vi "Main.vi"() -> ()   [LabVIEW 2018]
uses:
  States.ctl
panel:
  out "Minimalna waga pełnego akwarium":dbl format="%.2f"
  out "Współrzędne Y":dbl[](array[numeric]) format="%.2g"
  out "Współrzędne X":dbl[](array[numeric]) format="%.2g"
  out "Mocne punkty kompozycji":cluster{dbl[], dbl[]}(graph)
  out "Wykres pH wody w ciągu 23 dni":dbl[](graph)
  out "Waga pustego\n    akwarium":dbl format="%.2f"
  out "Rodzaje odczynów w\n       ciągu 23 dni":string[](array[string])
  out "Objętość brutto":dbl format="%.2g"
  out "Objętość netto":dbl format="%.2g"
  out "Wymagana ilość wody":dbl format="%.2g"
  out "pH wody w ciągu 23 dni":dbl[](array[numeric]) format="%.2f"
  in  "Wysokość":dbl=100.0 min=0.0
  in  "Długość":dbl=50.0 min=0.0
  in  "Szerokość":dbl=50.0 min=0.0
  in  "Grubość szyby":dbl=8.0 min=0.0
  in  "Zatrzymaj program":bool
  in  "Rysuj wykres mocnych punktów":bool
  in  "Policz wagę pustego\n        akwarium":bool
  in  "Rozpocznij symulację":bool
  # "Informacje zwrotne"
  # "Wprowadź dane \ndotyczące akwarium"
  # "l"
  # "cm"
  # "l"
  # "cm"
  # "l"
  # "cm"
  # "mm"
  # "kg"
  # "kg"
  # "Współrzędne punktów"
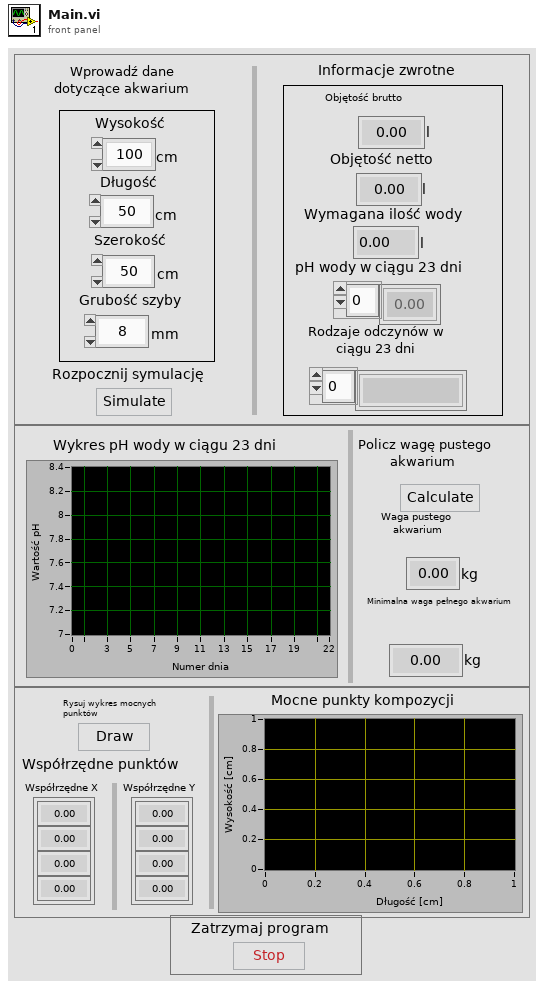
[diagram p1: front panel]
types:
  T1 = typedef "States.ctl" = enum16{"Init", "Idle", "Stop", "Simulate", "Calculate", "Draw"}
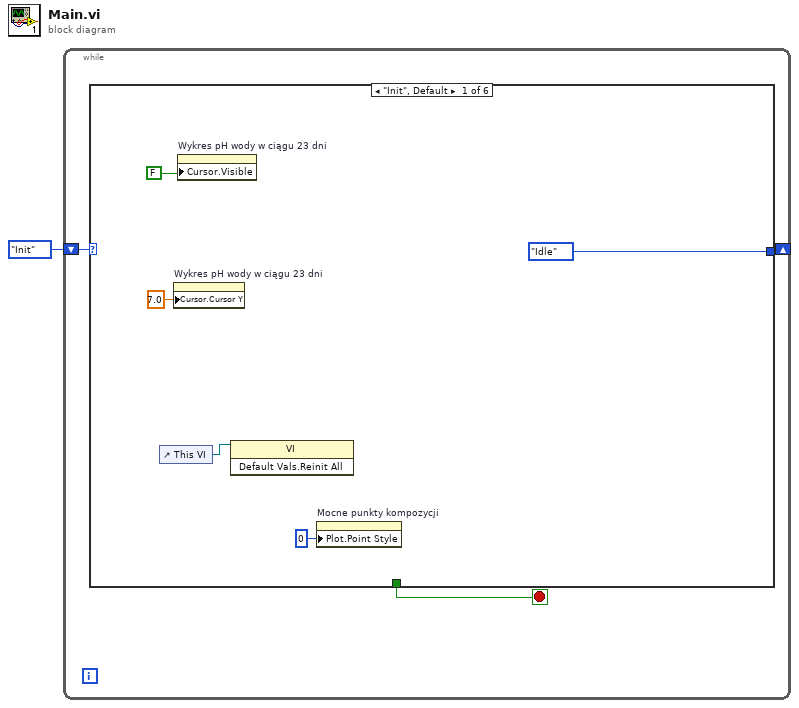
[diagram p0: block diagram]
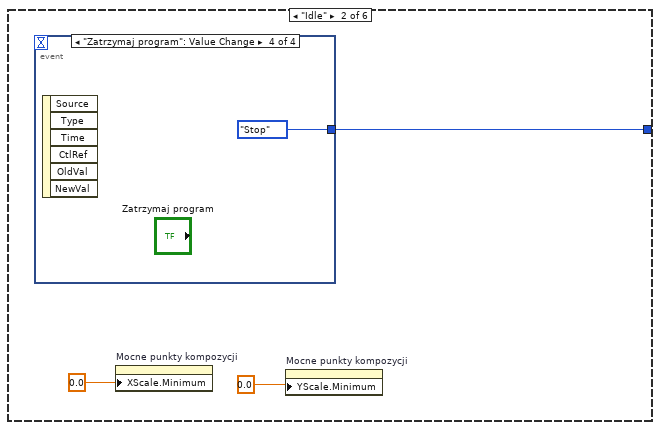
[diagram p2: hidden frame]
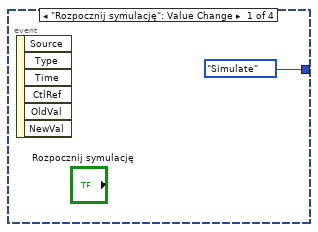
[diagram p3: hidden frame]
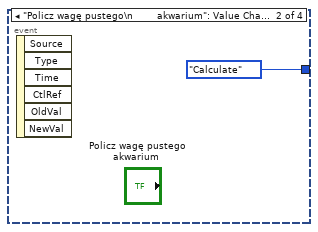
[diagram p4: hidden frame]
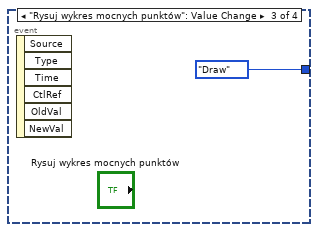
[diagram p5: hidden frame]
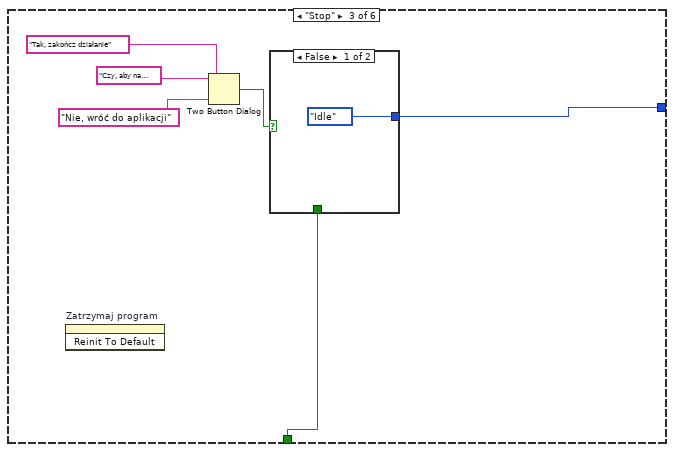
[diagram p6: hidden frame]
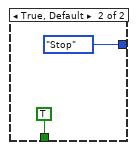
[diagram p7: hidden frame]
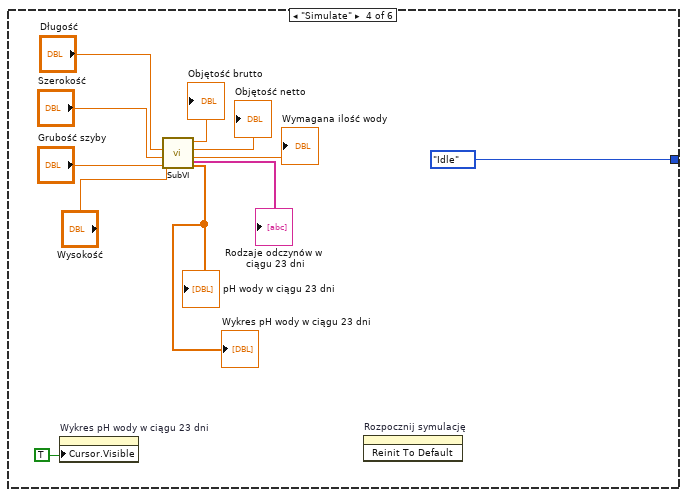
[diagram p8: hidden frame]
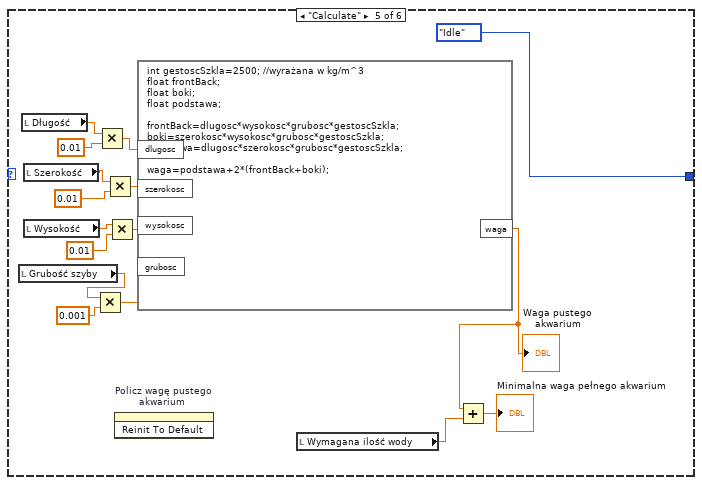
[diagram p9: hidden frame]
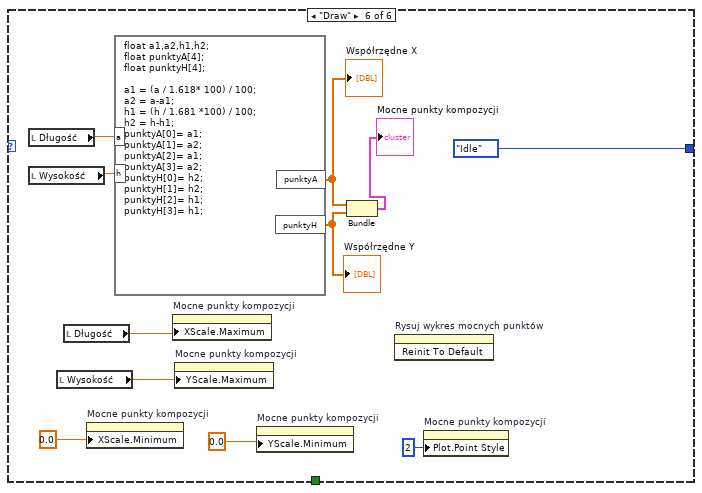
[diagram p10: hidden frame]
diagram:
  n1 = while {
    shift-right: [w2] -> _
    shift-left: States."Init" -> [w4]
    stop <- w3 stop-if-true
    n2 = case shown="\"Init\", Default" w4 {
      tunnel: [_ _ w18 _ _ _] -> w3
      tunnel: [States."Idle" w12 w17 States."Idle" States."Idle" States."Idle"] -> w2
      frame "Init", Default {
        n3 = control-ref of="This VI"() -> (w7:refnum<vi>)
        n4 = property on="Wykres pH wody w ciągu 23 dni" class="WFGraph (strict)"("Cursor.Cursor Y"=7.0 ("Cursor.Cursor Position:Cursor Y")) -> ()  [unwired: 2 in, 2 out]
        n5 = property on="Wykres pH wody w ciągu 23 dni" class="WFGraph (strict)"("Cursor.Visible"=FALSE) -> ()  [unwired: 2 in, 2 out]
        n6 = invoke class="VI" method="Default Vals.Reinit All"(reference=w7) -> ()  [unwired: 2 in, 3 out]
        n7 = property on="Mocne punkty kompozycji" class="XYGraph (strict)"("Plot.Point Style"=u8 0) -> ()  [unwired: 2 in, 2 out]
      }
      frame "Idle" {
        n8 = event shown="[3] \"Zatrzymaj program\": Value Change" {
          selector: _ -> [_ _ _ _]
          dyn-events: _ -> [_ _ _ _]
          timeout: _ -> [_ _ _ _]
          tunnel: [States."Simulate" States."Calculate" States."Draw" States."Stop"] -> w12
          event "Rozpocznij symulację": Value Change {
            n9 = event-data() -> ()  [unwired: 1 in, 6 out]
          }
          event "Policz wagę pustego\n        akwarium": Value Change {
            n10 = event-data() -> ()  [unwired: 1 in, 6 out]
          }
          event "Rysuj wykres mocnych punktów": Value Change {
            n11 = event-data() -> ()  [unwired: 1 in, 6 out]
          }
          event "Zatrzymaj program": Value Change {
            n12 = event-data() -> ()  [unwired: 1 in, 6 out]
          }
        }
        n13 = property on="Mocne punkty kompozycji" class="XYGraph (strict)"("XScale.Minimum"=0.0) -> ()  [unwired: 2 in, 2 out]
        n14 = property on="Mocne punkty kompozycji" class="XYGraph (strict)"("YScale.Minimum"=0.0) -> ()  [unwired: 2 in, 2 out]
      }
      frame "Stop" {
        n15 = invoke on="Zatrzymaj program" class="Bool" method="Reinit To Default"() -> ()  [unwired: 3 in, 3 out]
        n16 = Two Button Dialog(message="Czy, aby na pewno chcesz zakończyć działanie aplikacji?", 1:"Nie, wróć do aplikacji" ("F button name (\"Cancel\")"), 2:"Tak, zakończ działanie" ("T button name (\"OK\")")) -> (T button?=w19:bool)
        n17 = case shown="False" w19 {
          tunnel: [_ TRUE] -> w18
          tunnel: [States."Idle" States."Stop"] -> w17
          frame False {
          }
          frame True, Default {
          }
        }
      }
      frame "Simulate" {
        n18 = property on="Wykres pH wody w ciągu 23 dni" class="WFGraph (strict)"("Cursor.Visible"=TRUE) -> ()  [unwired: 2 in, 2 out]
        n19 = call "SubVI.vi"("Grubość szyby"="Grubość szyby", "Szerokość"="Szerokość", "Długość"="Długość", "Wysokość"="Wysokość") -> ("pH wody w ciągu 23 dni"=→"pH wody w ciągu 23 dni" →"Wykres pH wody w ciągu 23 dni":dbl[], "Wymagana ilość wody"=→"Wymagana ilość wody":dbl, "Objętość netto"=→"Objętość netto":dbl, "Objętość brutto"=→"Objętość brutto":dbl, "Rodzaje odczynów w\n       ciągu 23 dni"=→"Rodzaje odczynów w\n       ciągu 23 dni":string[])  [unwired: 3 in]
        n20 = invoke on="Rozpocznij symulację" class="Bool" method="Reinit To Default"() -> ()  [unwired: 3 in, 3 out]
      }
      frame "Calculate" {
        n21 = local read "Grubość szyby"() -> (w42:dbl)
        n22 = local read "Długość"() -> (w52:dbl)
        n23 = local read "Szerokość"() -> (w48:dbl)
        n24 = local read "Wysokość"() -> (w45:dbl)
        n25 = Multiply(x=w42, y=0.001) -> (x*y=w43:dbl)
        n26 = Multiply(x=w52, y=0.01) -> (x*y=w50:dbl)
        n27 = Multiply(x=w48, y=0.01) -> (x*y=w47:dbl)
        n28 = Multiply(x=w45, y=0.01) -> (x*y=w46:dbl)
        n29 = invoke on="Policz wagę pustego\n        akwarium" class="Bool" method="Reinit To Default"() -> ()  [unwired: 3 in, 3 out]
        n30 = formula code="int gestoscSzkla=2500; //wyrażana w kg/m^3\nfloat frontBack;\nfloat boki;\nfloat podstawa;\n\nfrontBack=dlugosc*wysokosc*grubosc*gestoscSzkla;\nboki=szerokosc*wysokosc*grubosc*gestoscSzkla;\npodstawa=dlugosc*szerokosc*grubosc*gestoscSzkla;\n\nwaga=podstawa+2*(frontBack+boki);"("dlugosc"=w50, "szerokosc"=w47, "wysokosc"=w46, "grubosc"=w43) -> ("waga"=w38:dbl)
        "Waga pustego\n    akwarium" <- w38
        n31 = local read "Wymagana ilość wody"() -> (w39:dbl)
        n32 = Add(x=w38, y=w39) -> (x+y=→"Minimalna waga pełnego akwarium":dbl)
      }
      frame "Draw" {
        n33 = local read "Długość"() -> (w62:dbl)
        n34 = local read "Wysokość"() -> (w61:dbl)
        n35 = local read "Wysokość"() -> (w56:dbl)
        n36 = local read "Długość"() -> (w57:dbl)
        n37 = property on="Mocne punkty kompozycji" class="XYGraph (strict)"("XScale.Minimum"=0.0) -> ()  [unwired: 2 in, 2 out]
        n38 = formula code="float a1,a2,h1,h2;\nfloat punktyA[4];\nfloat punktyH[4];\n\na1 = (a / 1.618* 100) / 100;\na2 = a-a1;\nh1 = (h / 1.681 *100) / 100;\nh2 = h-h1;\npunktyA[0]= a1;\npunktyA[1]= a2;\npunktyA[2]= a1;\npunktyA[3]= a2;\npunktyH[0]= h2;\npunktyH[1]= h2;\npunktyH[2]= h1;\npunktyH[3]= h1;"("a"=w62, "h"=w61) -> ("punktyA"=w60:dbl[], "punktyH"=w59:dbl[])
        "Współrzędne X" <- w60
        "Współrzędne Y" <- w59
        n39 = property on="Mocne punkty kompozycji" class="XYGraph (strict)"("XScale.Maximum"=w57) -> ()  [unwired: 2 in, 2 out]
        n40 = property on="Mocne punkty kompozycji" class="XYGraph (strict)"("YScale.Maximum"=w56) -> ()  [unwired: 2 in, 2 out]
        n41 = property on="Mocne punkty kompozycji" class="XYGraph (strict)"("YScale.Minimum"=0.0) -> ()  [unwired: 2 in, 2 out]
        n42 = Bundle(w60, w59) -> (→"Mocne punkty kompozycji":cluster{dbl[], dbl[]})  [unwired: 1 in]
        n43 = invoke on="Rysuj wykres mocnych punktów" class="Bool" method="Reinit To Default"() -> ()  [unwired: 3 in, 3 out]
        n44 = property on="Mocne punkty kompozycji" class="XYGraph (strict)"("Plot.Point Style"=u8 2) -> ()  [unwired: 2 in, 2 out]
      }
    }
  }
